vi "Event Handler.vi"(0 "Monkey in":refnum<class "Monkey.lvclass">, 5 "Event type":T1=enum."Message", 7 "Item Name":string, 9 "Data":variant, 11 "error in (no error)":errorcluster) -> (4 "Monkey out":refnum<class "Monkey.lvclass">, 15 "error out":errorcluster)   [LabVIEW 2020, in "Monkey.lvlib" / "Monkey.lvclass"]
doc: "This VI is the event handler of the uService: every time an event is triggered to the uService, this VI is called.\nNote: here you can access the Actor/Class data, but it will be the one coming out from Init. You cannot modify the values.\nThree different events are supported:\nI) Button Pressed: get called on a GUI button pressed. Item Name is the name (label) of the button, Data is empty.\nII) Shared Variable Updated: get called when a SV you subscribed to is updated. Item Name is the name of the SV, and Data is the value (note: you need to convert it to the proper type).\nIII) Message: get called every time a user event is generated using Send Message to Event Handler. The values of Item Name and Data are the one given to the Send Message to Event Handler.\nIV) Ready to launch?: this frame get called every time a new Run is initiated. Each uService is responsible of performing a self check before giving back the green light for the Run to start."
uses:
  Monkey.lvclass
  C:/Users/marco/Documents/GitHub_Lab/TALOS/talos/Father of all uServices/Father of all uServices/Father of all uServices.lvclass
  Father of all uServices/Father of all uServices/Event Handler Items.ctl
  Ancestor/Ancestor/Ancestor.lvclass/Ancestor.ctl
  Monkey Consumer Case Selector.ctl
  Father of all uServices/Father of all uServices Messages/Consumer Msg/Consumer Msg.lvclass/Consumer Msg.ctl
  Run Utilities/TypeDefs/Messages/Schedule Message.ctl
  Run Utilities/TypeDefs/DAQ Control.ctl
  Run Utilities/Schedule/Schedule.lvclass
  Run Utilities/TypeDefs/Script Checker Result.ctl
  Inner stop message.ctl
  Father of all uServices/Father of all uServices/Father of all uServices.lvclass/Father of all uServices.ctl
  FGV/Error Memory/Get Error Description.vi
  Support VIs/Get PC name.vi
  Ancestor/Ancestor/Read ID.vi
  Support VIs/Get Class Name.vi
  <vilib>/Utility/error.llb/Clear Errors.vi
  Father of all uServices/Father of all uServices Messages/Consumer Msg/Send Consumer.vi
  FGV/Error Memory/Error Memory Core.vi
  <vilib>/AdvancedString/Delimited String to 1D String Array.vi
  Support VIs/Circus Root Path.vi
  FGV/Error Memory/Error Crt Lvl checker.vi
  FGV/Error Memory/Error Memory Core.vi/40c8088d-b597-4017-91af-faa98e00292e.vi
  FGV/Error Memory/Error Memory Core.vi/d4a3ab98-063c-4e44-b43d-fbdcfe6c2be2.vi
  Father of all uServices/Father of all uServices/Father of all uServices.lvclass
  C:/Users/marco/Documents/GitHub_Lab/TALOS/builds/Actor Framework PPL/Actor Framework.lvlibp/1abvi3w/vi.lib/ActorFramework/Actor/Actor.lvclass
  Support VIs/Global Memory.vi
  <vilib>/Utility/LVClass/Get LV Class Name.vi
  Support VIs/Is in Packed Library.vi
  Support VIs/TALOS Root path.vi
  Support VIs/Read CSV worksheet.vi
  Support VIs/Global Constants.vi
  <vilib>/Utility/error.llb/General Error Handler.vi
  builds/Actor Framework PPL/Actor Framework.lvlibp/1abvi3w/vi.lib/ActorFramework/Actor/Read Self Enqueuer.vi
  <userlib>/_OpenG.lib/lvdata/lvdata.llb/Get Strings from Enum__ogtk.vi
  builds/Actor Framework PPL/Actor Framework.lvlibp/1abvi3w/vi.lib/ActorFramework/Message Enqueuer/Enqueue.vi
  Support VIs/Error Log.vi
  Ancestor/Ancestor/Ancestor.lvclass
  <vilib>/Comparison/Equal/Equal Functor/Equal Functor.lvclass
  Father of all uServices/Father of all uServices Messages/Consumer Msg/Consumer Msg.lvclass
  Run Utilities/Run Block/Run Block.lvclass
  Run Utilities/Run Utilities.lvlib
  TALOS.lvlib
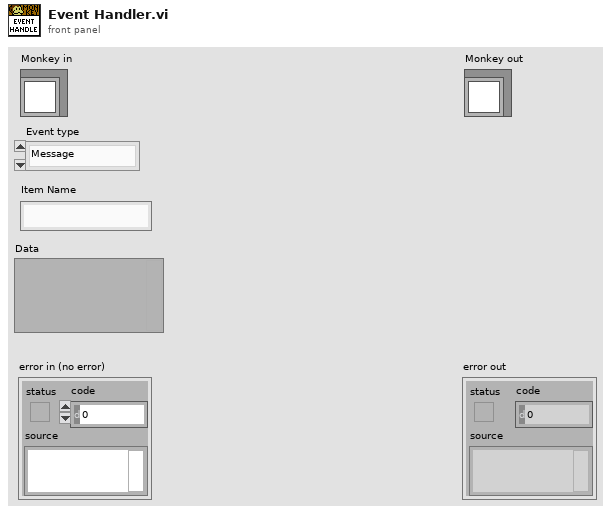
[diagram p1: front panel]
types:
  T1 = typedef "TALOS.lvlib/Father of all uServices.lvlib/Father of all uServices.lvclass/Event Handler Items.ctl" = enum16{"Button Pressed", "Shared Variable Updated", "Message", "Ready to launch?", "Safe Mode", "Start RUN", "Stop RUN"}
  T2 = typedef "Monkey.lvlib/Monkey.lvclass/Monkey Consumer Case Selector.ctl" = enum16{"Init", "Update GUI", "New schedule", "Check Script", "Submit Script", "Banana arrived", "Optimiser - evaluate RUN", "Optimiser - update RUN", "Quality Check", "What to do next", "Update Crit Lvl", "Skip Run", "Stop Schedule", "Skip schedule"}
  T3 = typedef "TALOS.lvlib/Run Utilities.lvlib/Schedule Message.ctl" = cluster{"uS Name":string, "Synchronised":bool, "DAQ Control":T4, "Schedule":refnum<class "Schedule.lvclass">}
  T4 = typedef "TALOS.lvlib/Run Utilities.lvlib/DAQ Control.ctl" = enum16{"On", "Off", "External"}
  T5 = typedef "TALOS.lvlib/Run Utilities.lvlib/Script Checker Result.ctl" = enum16{"Passed", "Failed", "Empty"}
  T6 = typedef "Monkey.lvlib/Monkey.lvclass/Inner stop message.ctl" = cluster{"Old value":bool, "Gracefully?":bool}
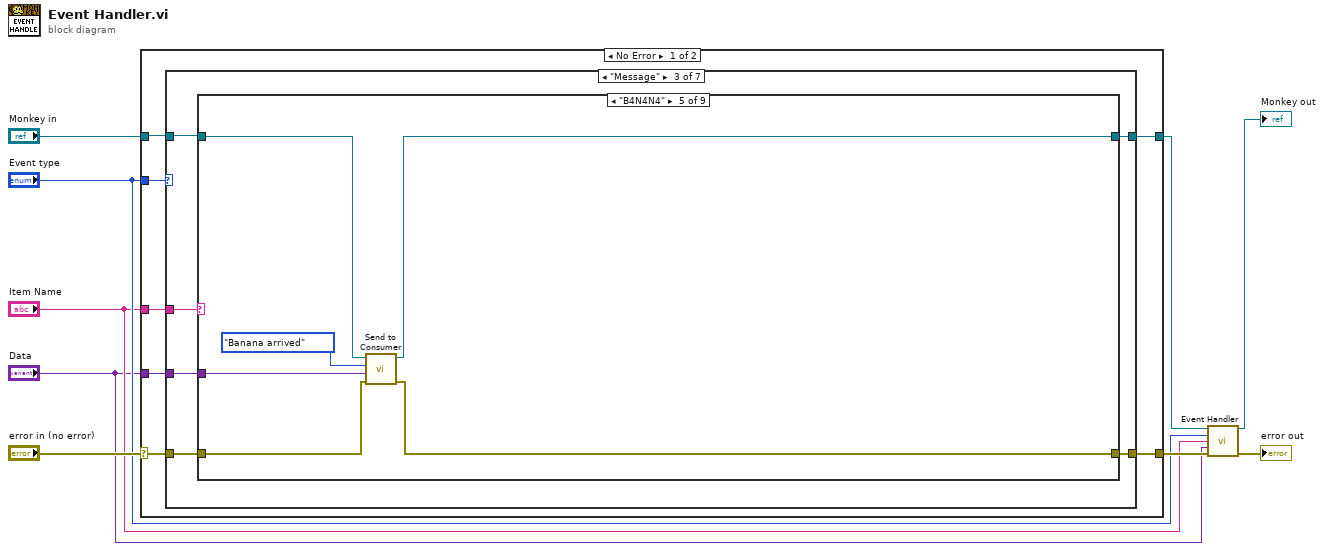
[diagram p0: block diagram]
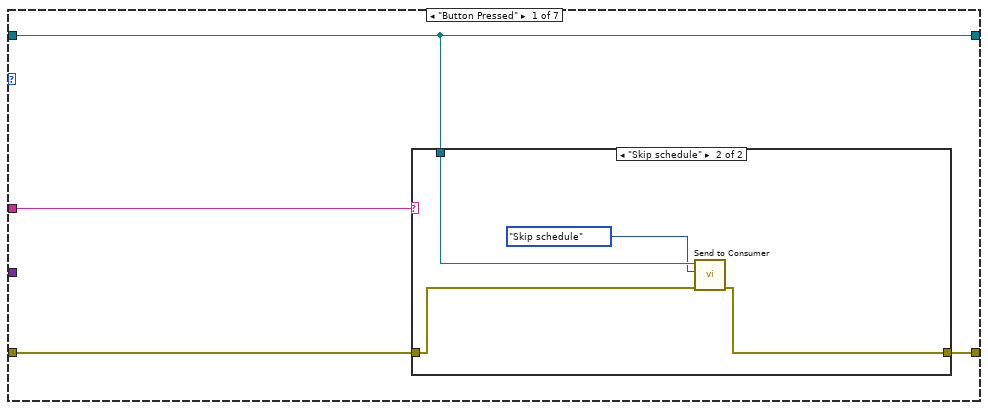
[diagram p2: hidden frame]
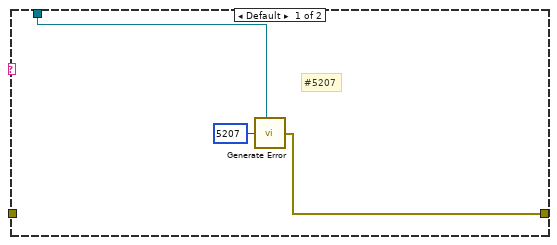
[diagram p3: hidden frame]
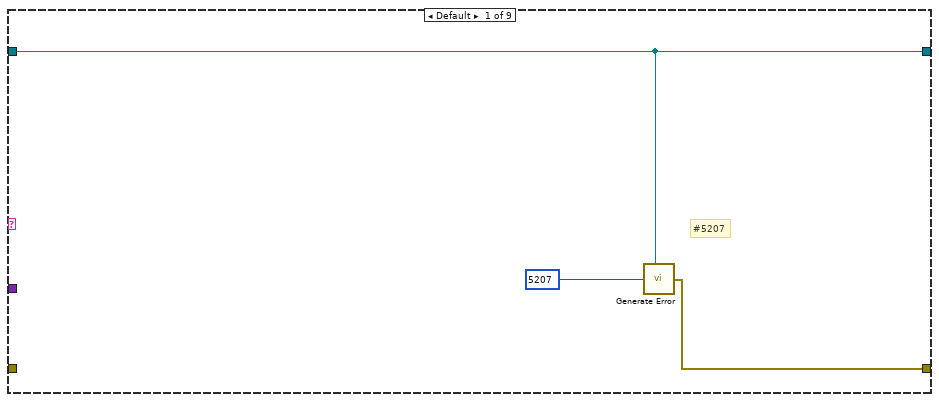
[diagram p5: hidden frame]
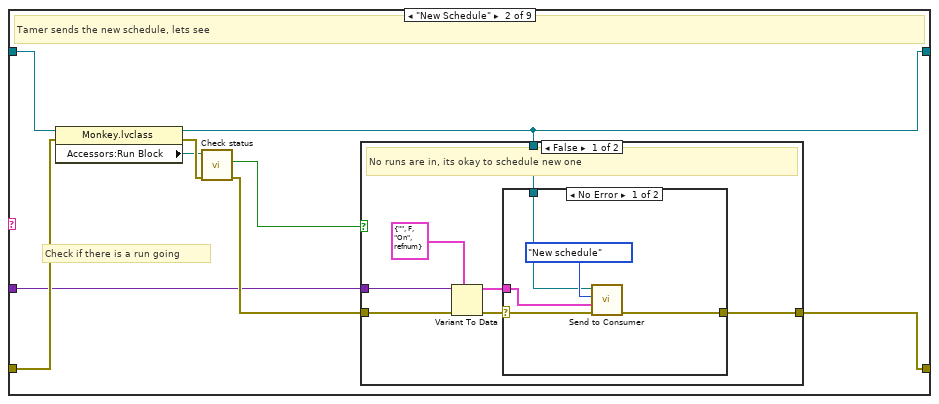
[diagram p6: hidden frame]
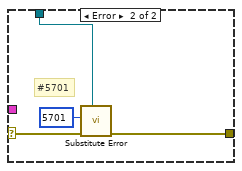
[diagram p7: hidden frame]
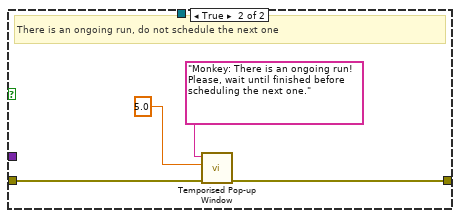
[diagram p8: hidden frame]
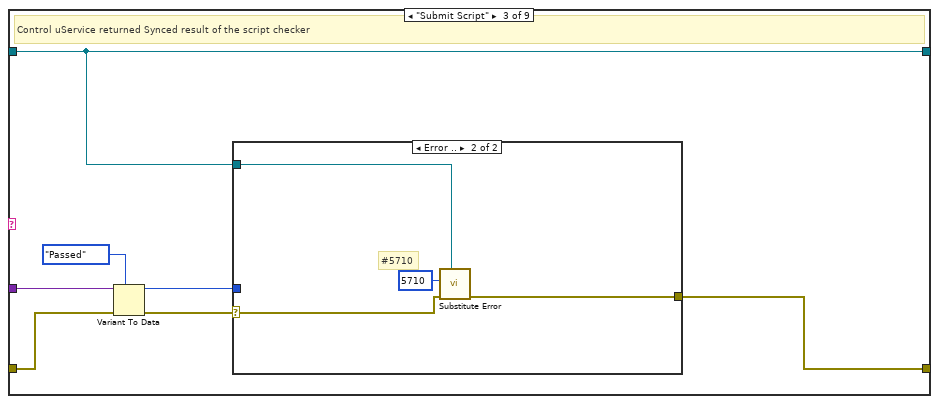
[diagram p9: hidden frame]
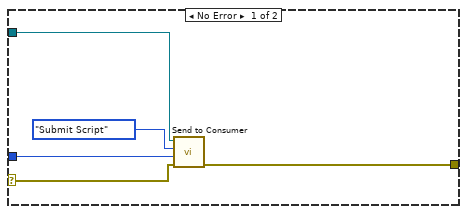
[diagram p10: hidden frame]
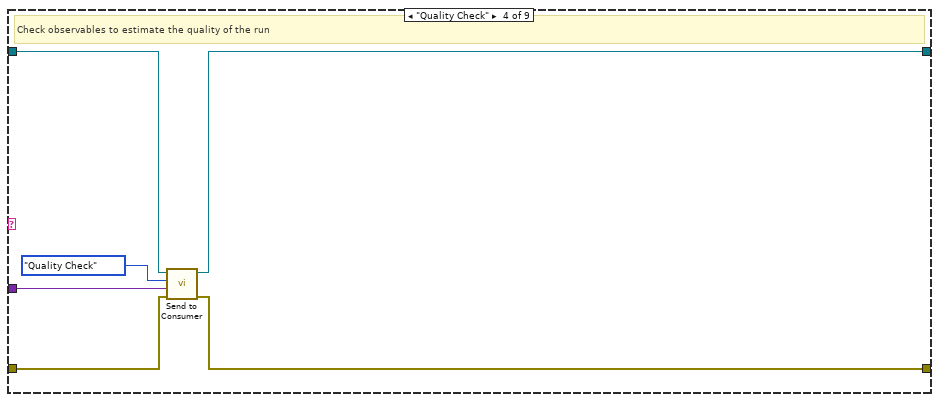
[diagram p11: hidden frame]
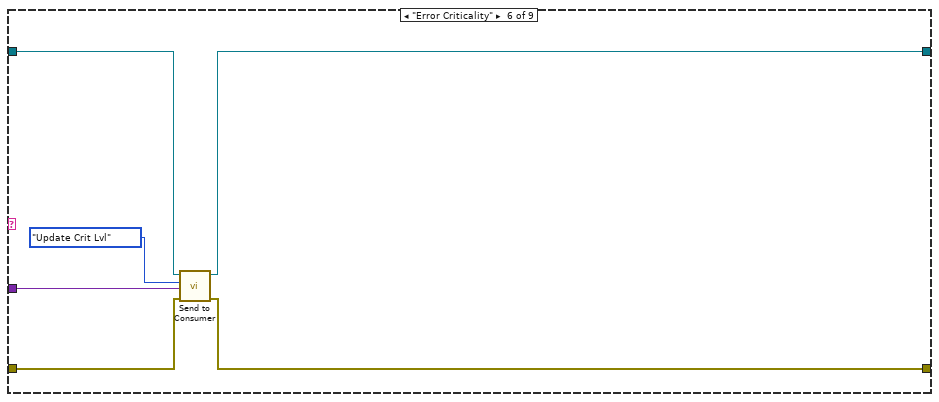
[diagram p12: hidden frame]
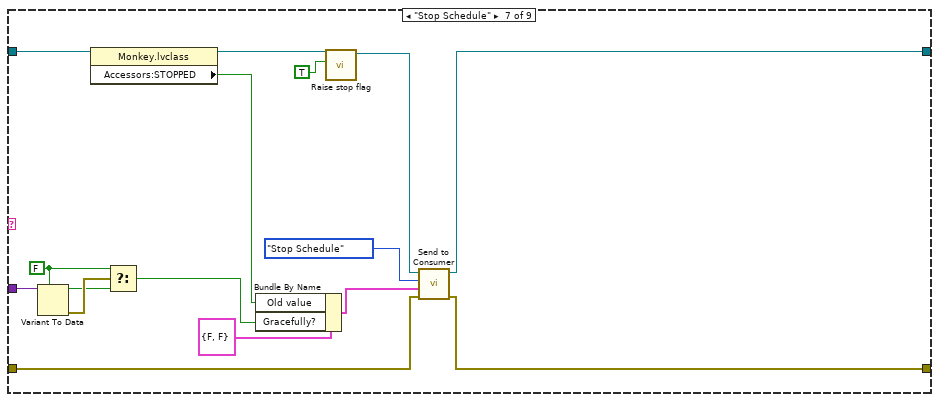
[diagram p13: hidden frame]
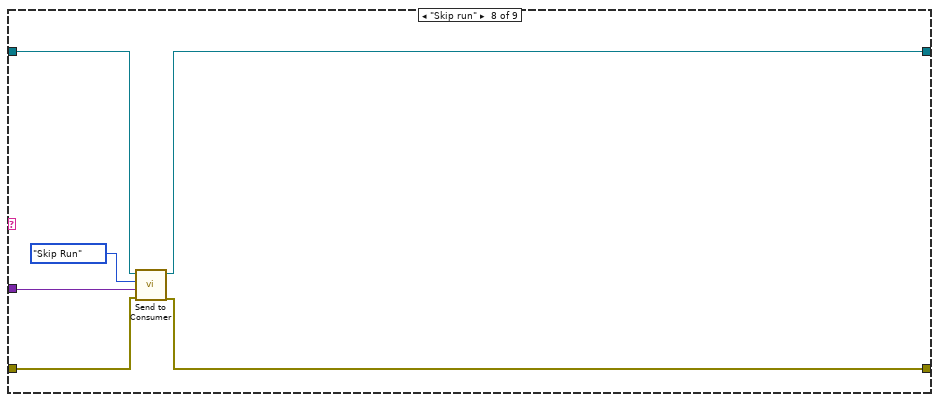
[diagram p14: hidden frame]
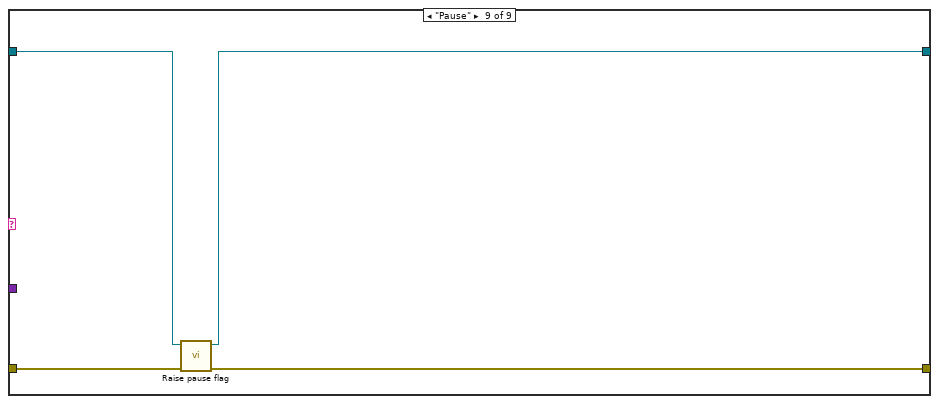
[diagram p15: hidden frame]
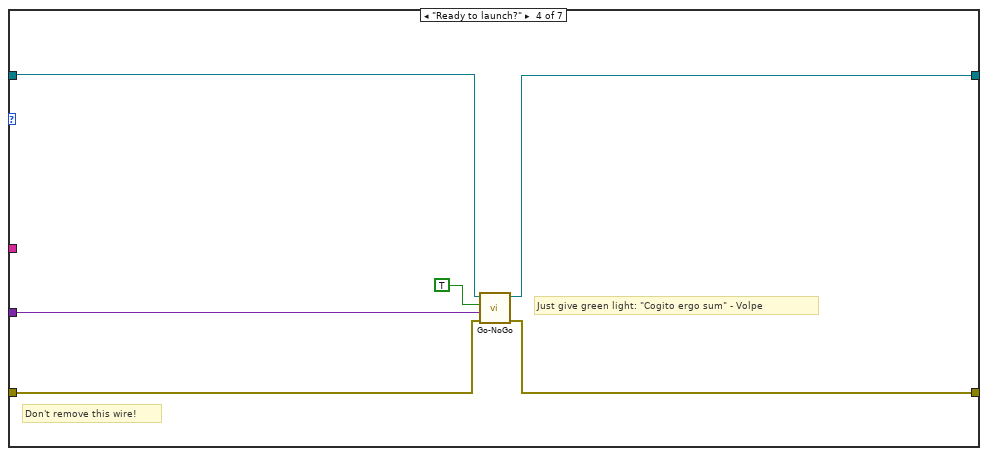
[diagram p16: hidden frame]
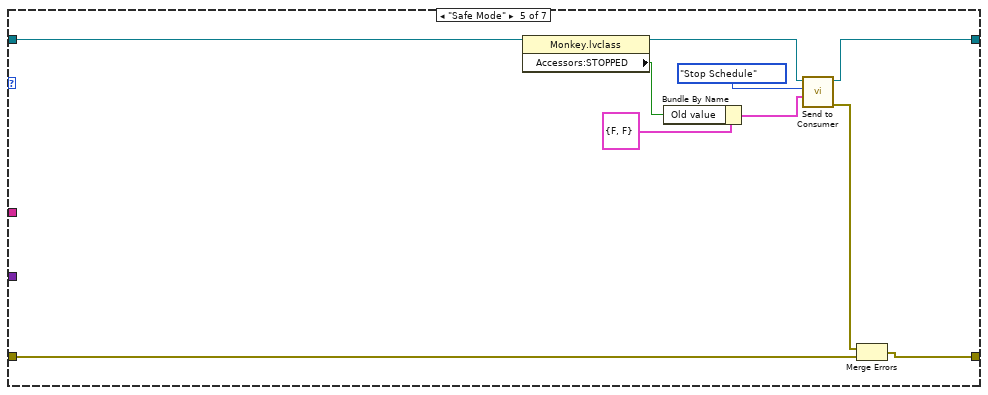
[diagram p17: hidden frame]
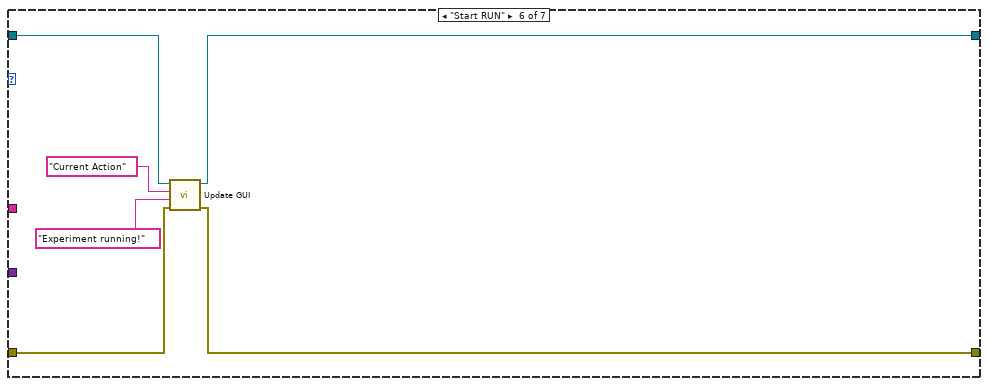
[diagram p18: hidden frame]
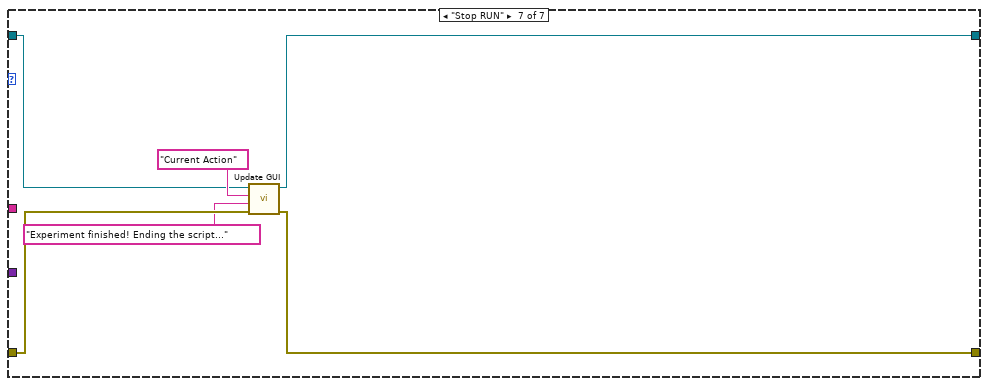
[diagram p19: hidden frame]
diagram:
  n1 = case shown="No Error" "error in (no error)" {
    selector: "error in (no error)" -> [w14 w157]
    tunnel: [w15 w157] -> w7
    tunnel: [w11 w156] -> w4
    tunnel: "Monkey in" -> [w10 w156]
    tunnel: "Event type" -> [w16 _]
    tunnel: "Item Name" -> [w13 _]
    tunnel: "Data" -> [w12 _]
    frame No Error {
      n2 = case shown="\"Message\"" w16 {
        tunnel: [w20 w29 w31 w132 w141 w145 w152] -> w15
        tunnel: w14 -> [w18 w29 w35 w133 w143 w148 w155]
        tunnel: w13 -> [w19 _ w34 _ _ _ _]
        tunnel: w10 -> [w17 w28 w32 w131 w137 w149 w151]
        tunnel: w12 -> [_ _ w33 w129 _ _ _]
        tunnel: [w17 w28 w30 w128 w139 w144 w150] -> w11
        frame "Button Pressed" {
          n3 = case shown="\"Skip schedule\"" w19 {
            tunnel: w18 -> [_ w26]
            tunnel: [w21 w25] -> w20
            tunnel: w17 -> [w22 w27]
            frame Default {
              # "#5207"
              n4 = call "Generate Error.vi"("Class"=w22, "Error Code"=5207) -> ("error out"=w21:errorcluster)  [unwired: 5 in]
            }
            frame "Skip schedule" {
              n5 = call "Send to Consumer.vi"("error in (no error)"=w26, "Case ID"=Monkey_Consumer_Case_Selector."Skip schedule" ("Monkey Consumer Case Selector"), "uService Template in"=w27) -> ("error out"=w25:errorcluster)  [unwired: 7 in, 1 out]
            }
          }
        }
        frame "Shared Variable Updated" {
        }
        frame "Message" {
          n6 = case shown="\"B4N4N4\"" w34 {
            tunnel: w35 -> [_ w47 w73 w87 w94 w101 w117 w123 w126]
            tunnel: w33 -> [_ w44 w74 w89 w92 w100 w108 w122 _]
            tunnel: w32 -> [w36 w40 w68 w85 w91 w97 w114 w118 w127]
            tunnel: [w37 w43 w69 w86 w93 w99 w116 w121 w125] -> w31
            tunnel: [w36 w39 w68 w84 w90 w96 w113 w119 w124] -> w30
            frame Default {
              # "#5207"
              n7 = call "Generate Error.vi"("Class"=w36, "Error Code"=5207) -> ("error out"=w37:errorcluster)  [unwired: 5 in]
            }
            frame "New Schedule" {
              # "Check if there is a run going"
              # "Tamer sends the new schedule, lets see"
              n8 = property class="Monkey.lvclass"(reference=w40, error in=w47) -> (reference out=w39:refnum<class "Monkey.lvclass">, error out=w45:errorcluster, "Accessors:Run Block"=w42:refnum<class "Run Block.lvclass">)
              n9 = call-dynamic "Check status.vi"("error in (no error)"=w45, "Run Block in"=w42) -> ("error out"=w46:errorcluster, "Running"=w41:bool)  [unwired: 7 in, 1 out]
              n10 = case shown="False" w41 {
                tunnel: w44 -> [w54 _]
                tunnel: [w51 w64] -> w43
                tunnel: w39 -> [w50 _]
                tunnel: w46 -> [w49 w67]
                frame False {
                  # "No runs are in, its okay to schedule new one"
                  n11 = Variant To Data(error in=w49, type=T3 {"uS Name"="", "Synchronised"=FALSE, "DAQ Control"=enum."On", "Schedule"=refnum} ("Monkey Schedule Message"), Variant=w54) -> (data=w52:T3, error out=w53:errorcluster)
                  n12 = case shown="No Error" w53 {
                    selector: w53 -> [w57 w63]
                    tunnel: w52 -> [w56 _]
                    tunnel: w50 -> [w58 w60]
                    tunnel: [w55 w61] -> w51
                    frame No Error {
                      n13 = call "Send to Consumer.vi"("error in (no error)"=w57, "Data"=w56, "Case ID"=Monkey_Consumer_Case_Selector."New schedule" ("Monkey Consumer Case Selector"), "uService Template in"=w58) -> ("error out"=w55:errorcluster)  [unwired: 6 in, 1 out]
                    }
                    frame Error {
                      # "#5701"
                      n14 = call "Substitute Error.vi"("LabVIEW Object"=w60, "error in (no error)"=w63, "Error Code"=5701) -> ("error out"=w61:errorcluster)  [unwired: 8 in]
                    }
                  }
                }
                frame True {
                  # "There is an ongoing run, do not schedule the next one"
                  n15 = call "Temporised Pop-up Window.vi"("error in (no error)"=w67, "Timeout"=5.0, "Text"="Monkey: There is an ongoing run! Please, wait until finished before scheduling the next one.") -> ("error out"=w64:errorcluster)  [unwired: 8 in]
                }
              }
            }
            frame "Submit Script" {
              # "Control uService returned Synced result of the script checker"
              n16 = Variant To Data(error in=w73, type=Script_Checker_Result."Passed" ("Script Checker Result"), Variant=w74) -> (data=w70:T5, error out=w71:errorcluster)
              n17 = case shown="Error .." w71 {
                selector: w71 -> [w76 w81]
                tunnel: w70 -> [w78 _]
                tunnel: w68 -> [w77 w82]
                tunnel: [w75 w83] -> w69
                frame No Error {
                  n18 = call "Send to Consumer.vi"("error in (no error)"=w76, "Data"=w78, "Case ID"=Monkey_Consumer_Case_Selector."Submit Script" ("Monkey Consumer Case Selector"), "uService Template in"=w77) -> ("error out"=w75:errorcluster)  [unwired: 6 in, 1 out]
                }
                frame Error {
                  # "#5710"
                  n19 = call "Substitute Error.vi"("LabVIEW Object"=w82, "error in (no error)"=w81, "Error Code"=5710) -> ("error out"=w83:errorcluster)  [unwired: 8 in]
                }
              }
            }
            frame "Quality Check" {
              # "Check observables to estimate the quality of the run"
              n20 = call "Send to Consumer.vi"("error in (no error)"=w87, "Data"=w89, "Case ID"=Monkey_Consumer_Case_Selector."Quality Check" ("Monkey Consumer Case Selector"), "uService Template in"=w85) -> ("error out"=w86:errorcluster, "uService Template out"=w84:refnum<class "Monkey.lvclass">)  [unwired: 6 in]
            }
            frame "B4N4N4" {
              n21 = call "Send to Consumer.vi"("error in (no error)"=w94, "Data"=w92, "Case ID"=Monkey_Consumer_Case_Selector."Banana arrived" ("Monkey Consumer Case Selector"), "uService Template in"=w91) -> ("error out"=w93:errorcluster, "uService Template out"=w90:refnum<class "Monkey.lvclass">)  [unwired: 6 in]
            }
            frame "Error Criticality" {
              n22 = call "Send to Consumer.vi"("error in (no error)"=w101, "Data"=w100, "Case ID"=Monkey_Consumer_Case_Selector."Update Crit Lvl" ("Monkey Consumer Case Selector"), "uService Template in"=w97) -> ("error out"=w99:errorcluster, "uService Template out"=w96:refnum<class "Monkey.lvclass">)  [unwired: 6 in]
            }
            frame "Stop Schedule" {
              w109 = FALSE
              n23 = Variant To Data(type=w109, Variant=w108) -> (data=w110:bool, error out=w111:errorcluster)  [unwired: 1 in]
              n24 = property class="Monkey.lvclass"(reference=w114) -> (reference out=w104:refnum<class "Monkey.lvclass">, "Accessors:STOPPED"=w106:bool)  [unwired: 1 in, 1 out]
              n25 = Select(t=w109, s=w111, f=w110) -> (s? t:f=w107:bool)
              n26 = Bundle By Name(cluster=T6 {"Old value"=FALSE, "Gracefully?"=FALSE} ("Stop msg"), "Old value"=w106, "Gracefully?"=w107) -> (w105:T6)
              n27 = call-dynamic "Raise stop flag.vi"("on/off"=TRUE, "Monkey in"=w104) -> ("Monkey out"=w103:refnum<class "Monkey.lvclass">)  [unwired: 8 in, 1 out]
              n28 = call "Send to Consumer.vi"("error in (no error)"=w117, "Data"=w105, "Case ID"=Monkey_Consumer_Case_Selector."Stop Schedule" ("Monkey Consumer Case Selector"), "uService Template in"=w103) -> ("error out"=w116:errorcluster, "uService Template out"=w113:refnum<class "Monkey.lvclass">)  [unwired: 6 in]
            }
            frame "Skip run" {
              n29 = call "Send to Consumer.vi"("error in (no error)"=w123, "Data"=w122, "Case ID"=Monkey_Consumer_Case_Selector."Skip Run" ("Monkey Consumer Case Selector"), "uService Template in"=w118) -> ("error out"=w121:errorcluster, "uService Template out"=w119:refnum<class "Monkey.lvclass">)  [unwired: 6 in]
            }
            frame "Pause" {
              n30 = call-dynamic "Raise pause flag.vi"("error in (no error)"=w126, "Monkey in"=w127) -> ("error out"=w125:errorcluster, "Monkey out"=w124:refnum<class "Monkey.lvclass">)  [unwired: 8 in]
            }
          }
        }
        frame "Ready to launch?" {
          # "Don't remove this wire!"
          # "Just give green light: \"Cogito ergo sum\" - Volpe"
          n31 = call-dynamic "Go-NoGo.vi"("error in (no error)"=w133, "Go-NoGo Data"=w129, "Go?"=TRUE, "Father of all uServices in"=w131) -> ("error out"=w132:errorcluster, "Father of all uServices out"=w128:refnum<class "Monkey.lvclass">)  [unwired: 6 in]
        }
        frame "Safe Mode" {
          n32 = property class="Monkey.lvclass"(reference=w137) -> (reference out=w136:refnum<class "Monkey.lvclass">, "Accessors:STOPPED"=w135:bool)  [unwired: 1 in, 1 out]
          n33 = Bundle By Name(cluster=T6 {"Old value"=FALSE, "Gracefully?"=FALSE} ("Stop msg"), "Old value"=w135) -> (w134:T6)
          n34 = call "Send to Consumer.vi"("Data"=w134, "Case ID"=Monkey_Consumer_Case_Selector."Stop Schedule" ("Monkey Consumer Case Selector"), "uService Template in"=w136) -> ("error out"=w140:errorcluster, "uService Template out"=w139:refnum<class "Monkey.lvclass">)  [unwired: 7 in]
          n35 = Merge Errors(w140, w143) -> (w141:errorcluster)
        }
        frame "Start RUN" {
          n36 = call "Update GUI.vi"("error in (no error)"=w148, "Data"="Experiment running!" ("GUI Item Name"), "GUI Item Name"="Current Action", "uService Template in"=w149) -> ("error out"=w145:errorcluster, "uService Template out"=w144:refnum<class "Monkey.lvclass">)  [unwired: 6 in]
        }
        frame "Stop RUN" {
          n37 = call "Update GUI.vi"("error in (no error)"=w155, "Data"="Experiment finished! Ending the script..." ("GUI Item Name"), "GUI Item Name"="Current Action", "uService Template in"=w151) -> ("error out"=w152:errorcluster, "uService Template out"=w150:refnum<class "Monkey.lvclass">)  [unwired: 6 in]
        }
      }
    }
    frame Error {
    }
  }
  n38 = call-parent "Event Handler.vi"("uService Template in"=w4, "Event type"="Event type", "Item Name"="Item Name", "Data"="Data", "error in (no error)"=w7) -> ("uService Template out"=→"Monkey out":refnum<class "Monkey.lvclass">, "error out"=→"error out":errorcluster)  [unwired: 9 in]
